vi "1 - Write Temperature to ASCII File (Original).vi"() -> ()   [LabVIEW 2012]
panel:
  out "Alarm Output":bool
  in  "Alarm Level":dbl=26.0
  out "Temperature":dynamicdata(graph)
  in  "stop":bool
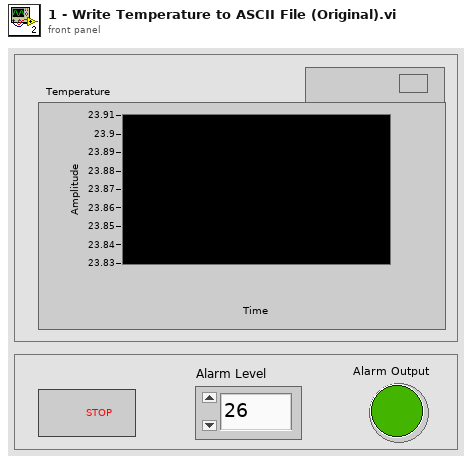
[diagram p1: front panel]
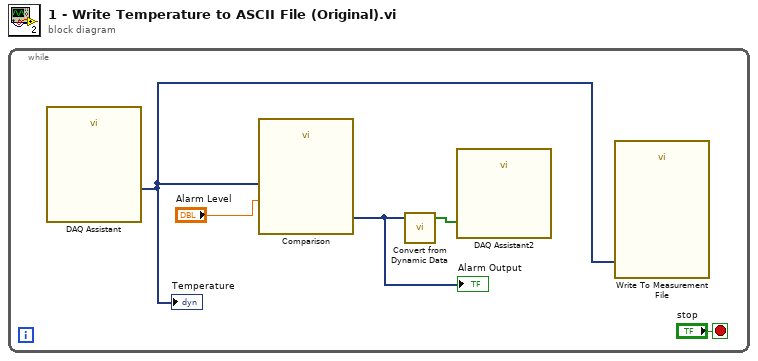
[diagram p0: block diagram]
diagram:
  n1 = while {
    stop <- "stop" stop-if-true
    n2 = call "DAQ Assistant"() -> ("data"=w3:dynamicdata)  [unwired: 6 in, 13 out]
    "Temperature" <- w3
    n3 = call "Comparison"("Operand 2"="Alarm Level", "Operand 1"=w3) -> ("Result"=w2:dynamicdata)  [unwired: 1 in, 8 out]
    "Alarm Output" <- w2
    n4 = call "Convert from Dynamic Data"("Dynamic Data Type"=w2) -> ("Array"=w1:bool[])  [unwired: 3 in]
    n5 = call "DAQ Assistant2"("data"=w1) -> ()  [unwired: 4 in, 15 out]
    n6 = call "Write To Measurement File"("Signals"=w3) -> ()  [unwired: 16 in, 3 out]
  }
